vi "GUI_Cameras_v1.2.0.vi"() -> ()   [LabVIEW 2011]
uses:
  <vilib>/Utility/miscctls.llb/LVRectTypeDef.ctl
panel:
  out "Zoom changed":bool
  out "Zoom old":cluster{"X":sgl, "Y":sgl}
  out "MaxCounts":dbl(slide) scale=0.0..256.0
  out "ratio(h)":bool=TRUE
  out "fixsize":bool
  out "Change Ratio":cluster{"X":sgl, "Y":sgl}={"X"=1.6671598, "Y"=0.6151203}
  out "old Panel Bounds":T1={"Left"=105, "Top"=80, "Right"=781, "Bottom"=662}
  in  "shotnumber":i32=354
  in  "gain":dbl
  in  "exposure":dbl=0.52 caption="Exposure"
  in  "save":bool
  in  "trigger":bool
  in  "triggerdelay":dbl
  out "error (h)":bool
  in  "Main Tap":enum32{"IMAQ", "Network", "Internal", "Array"}(tab)
  out "Image (IMAQ)":T2(plugin-control)
  out "local Port":u16=65401
  out "Remote Host":string="192.168.10.157"
  out "port or service name":u16=65400
  in  "timeout ms (slow resp)":i32=500
  in  "reset":bool
  out "All Devices (h)":string[](array[string])
  out "centroidy":dbl
  out "fast ID (h)":refnum<k16>
  out "slow ID (h)":refnum<k16>
  out "error out":errorcluster
  out "connections (hidden)":variant[](array[variant])=[variant(refnum<k16> refnum), variant(refnum<k16> refnum)]
  in  "time to wait (main loop)":i32=200
  in  "time to wait (TCP)":i32=10
  out "Data String":string="exposure,0.520000\r\ntrigger,off\r\nsave,off\r\ngain,0.000000\r\n"
  in  "send":bool
  in  "localsavingpath":path
  out "centroidy":dbl
  out "Image (array)":u8[][](graph)
  out "Device Name (h)":string="FakeCam1"
  out "stop":bool
  out "error message":string
  out "image connection":bool
  out "data connection ok":bool
  # "Data"
  # "Image"
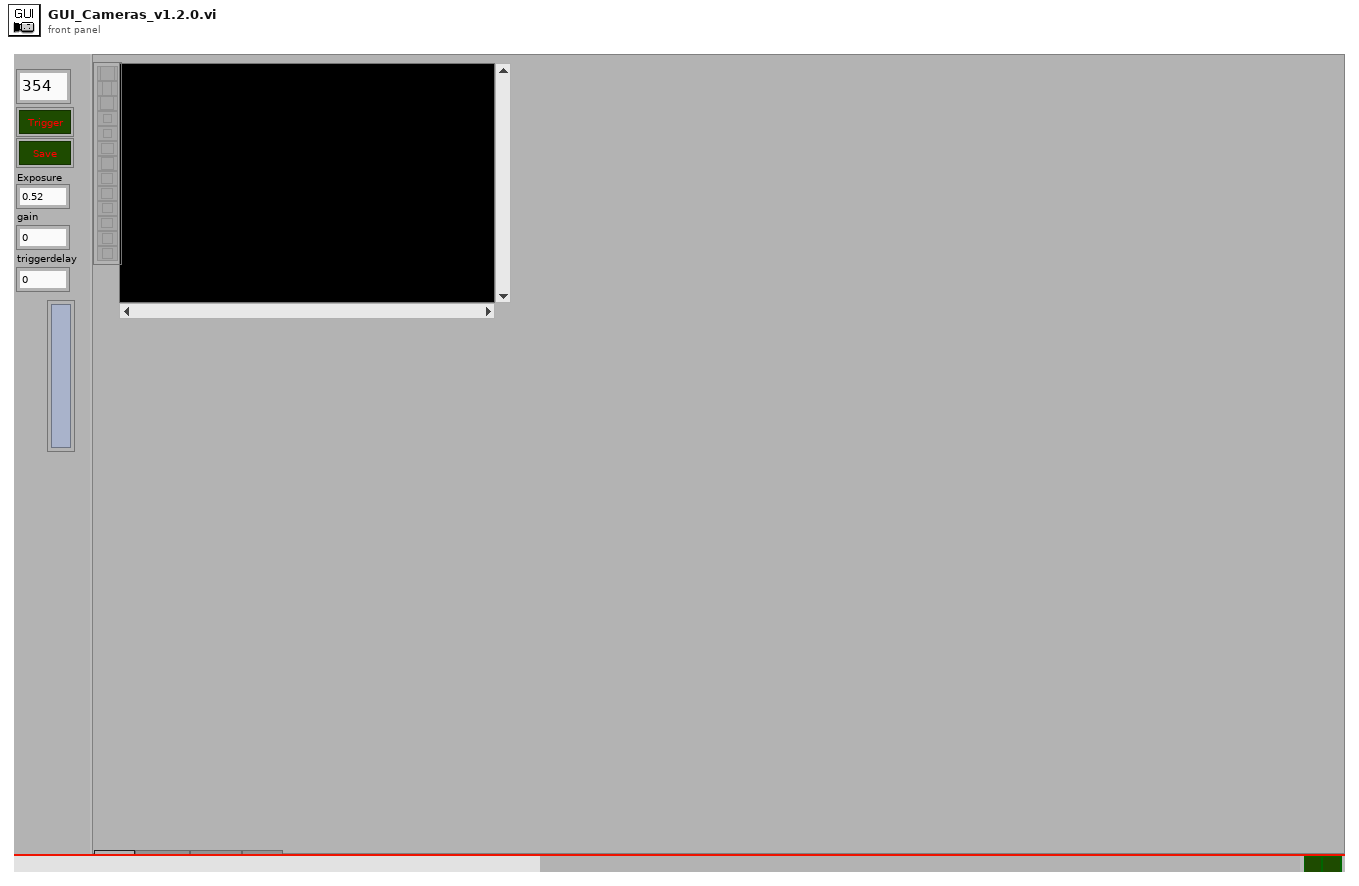
[diagram p1: front panel]
types:
  T1 = typedef "LVRectTypeDef.ctl" = cluster{"Left":i16, "Top":i16, "Right":i16, "Bottom":i16}
  T2 = typedef "IMAQ Image.ctl" = refnum<image>
  T3 = enum16{"Grayscale", "Binary", "Gradient", "Rainbow", "Temperature", "User Defined"}
  T4 = typedef "Image Type" = u32
  T5 = cluster{"Global Rectangle":i32[], "Contours":cluster{"Contour Type":u32, "ROI Type":u32, "Points":i32[]}[]}
  T6 = typedef "ROI Descriptor" = cluster{"Global Rectangle":i32[], "Contours":cluster{"ID":enum32{"External", "Internal"}, "Type":u32, "Coordinates":i32[]}[]}
  T7 = typedef "LVBoundsTypeDef.ctl" = cluster{"Width":u32, "Height":u32}
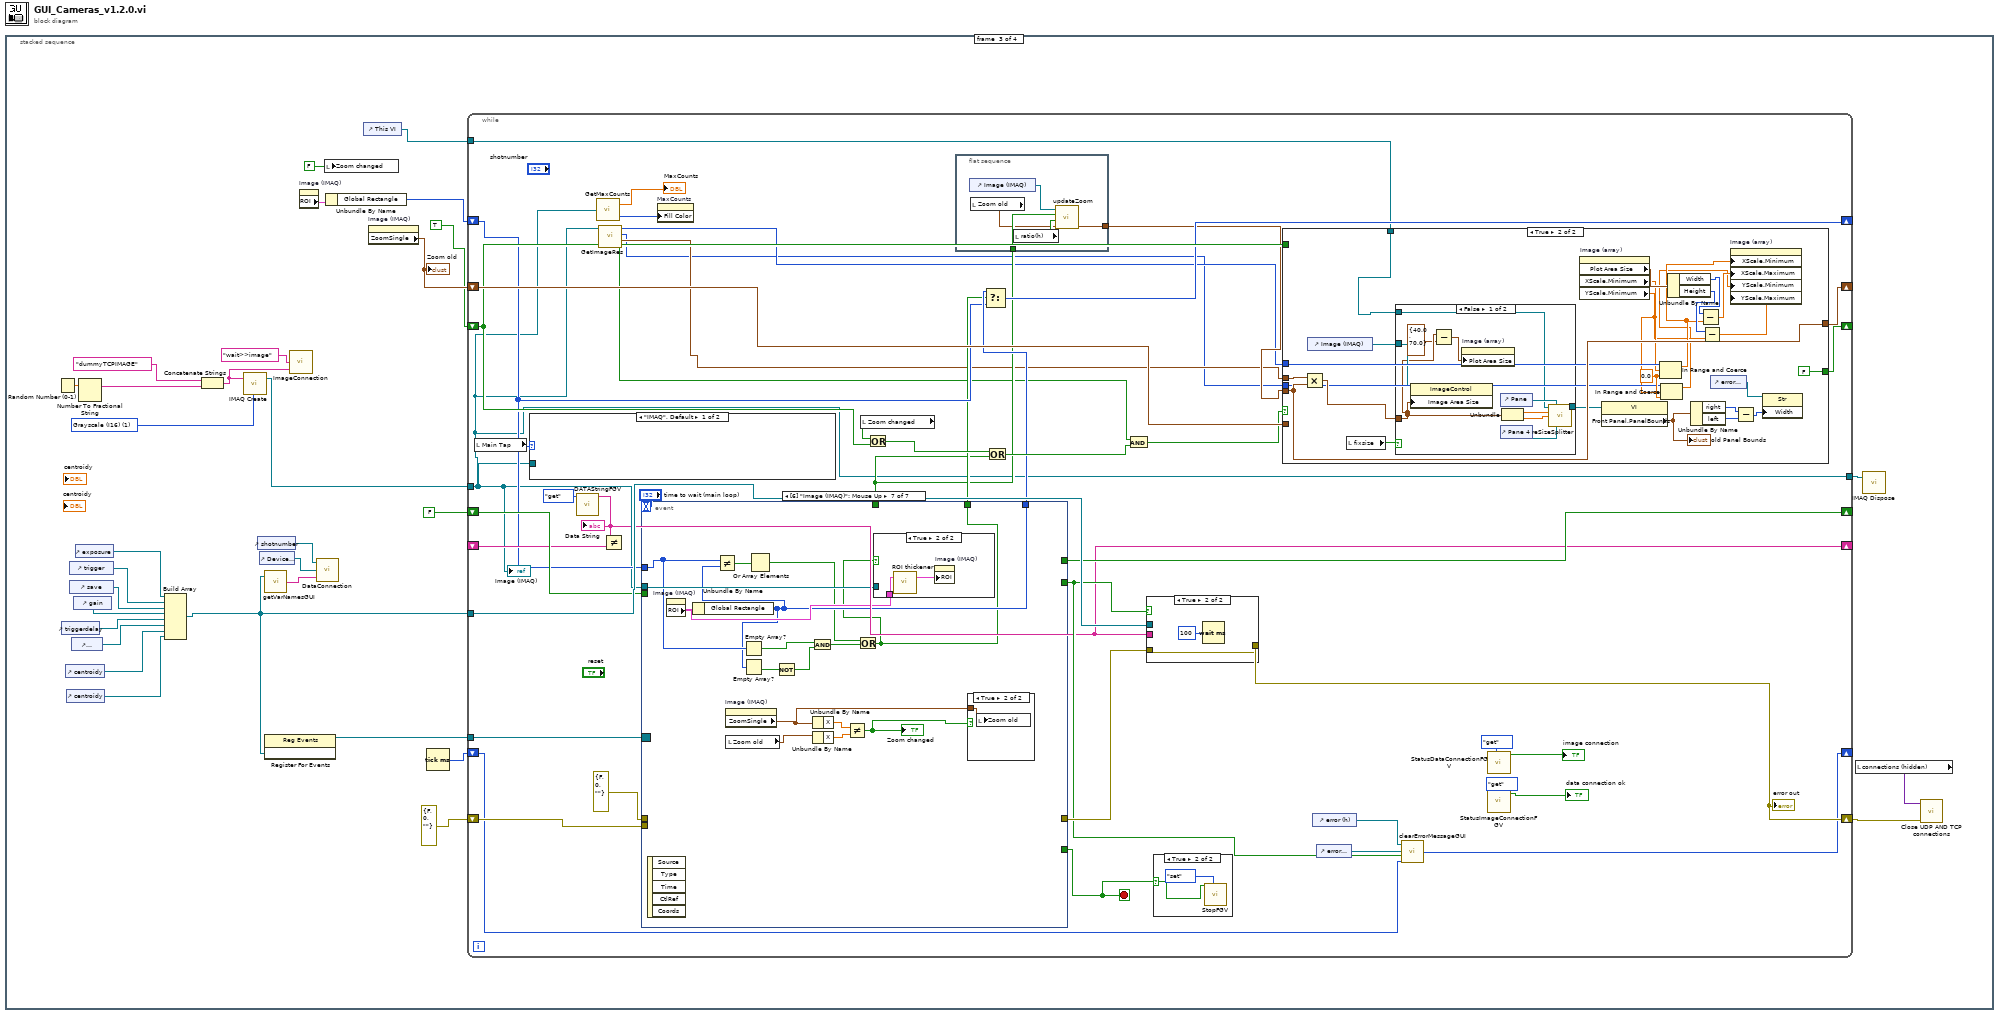
[diagram p0: block diagram]
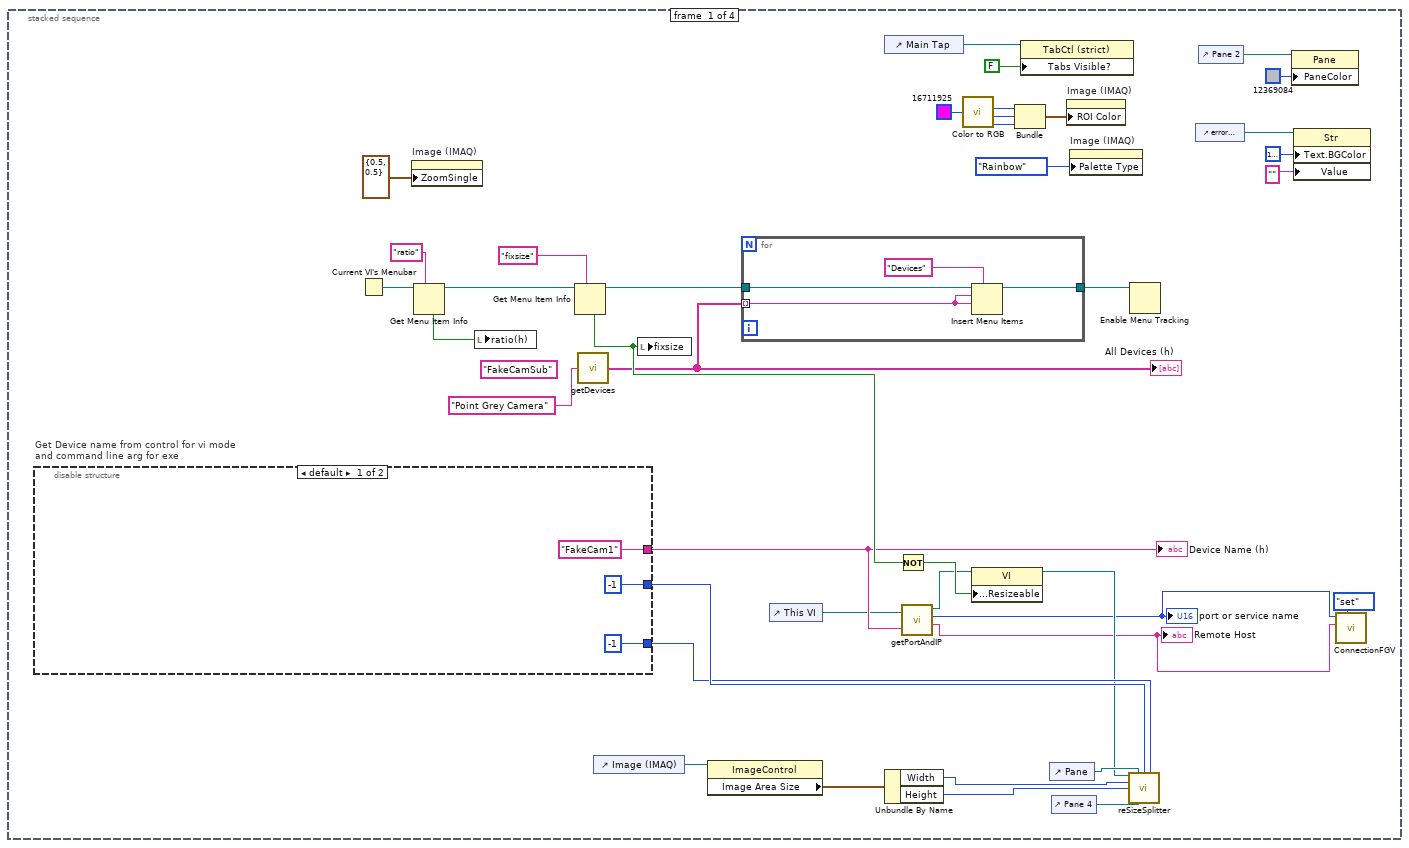
[diagram p2: hidden frame]
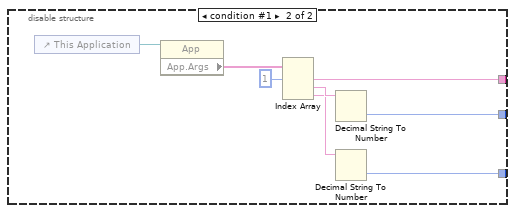
[diagram p3: hidden frame]
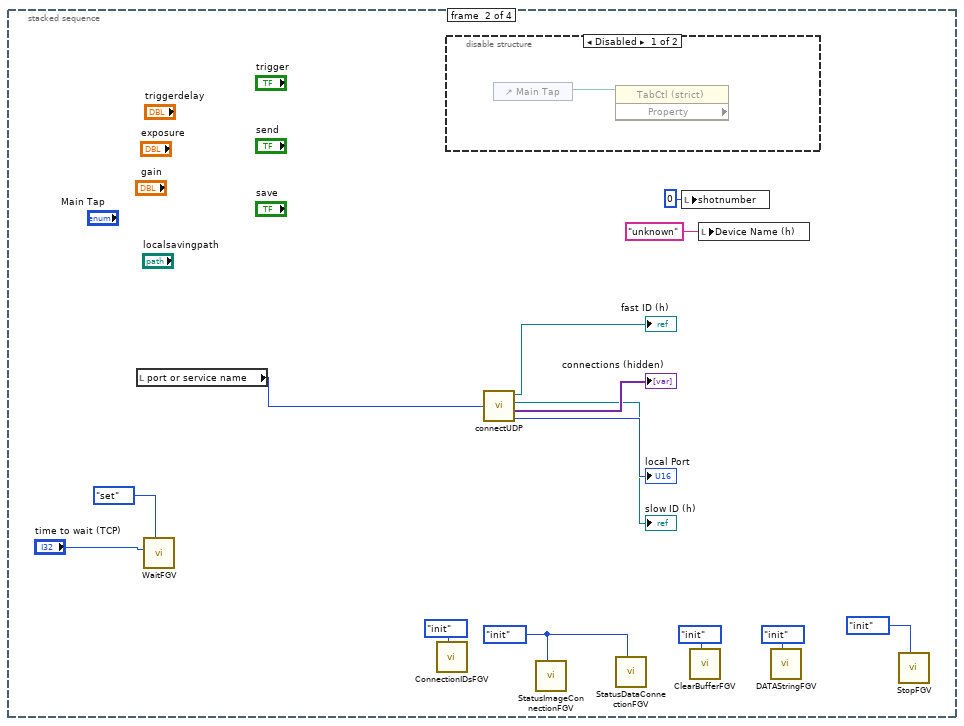
[diagram p4: hidden frame]
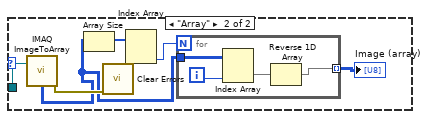
[diagram p7: hidden frame]
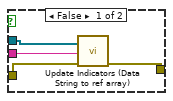
[diagram p10: hidden frame]
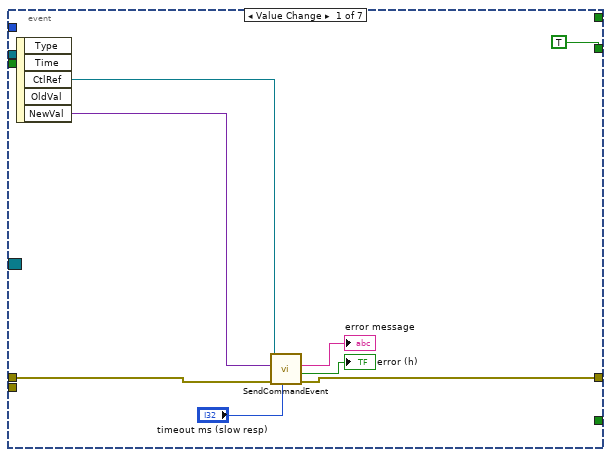
[diagram p11: hidden frame]
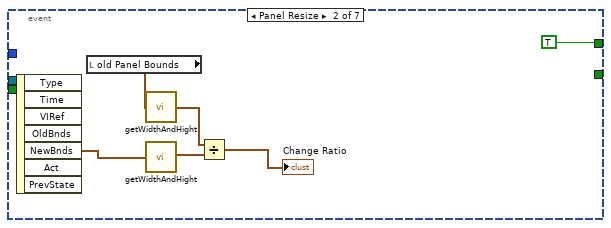
[diagram p12: hidden frame]
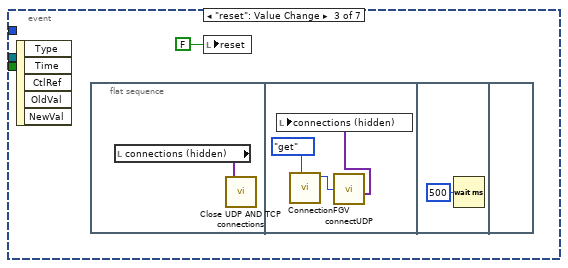
[diagram p13: hidden frame]
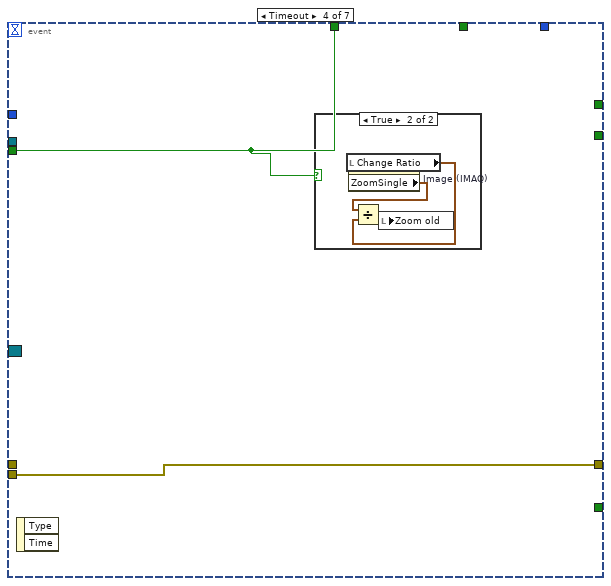
[diagram p14: hidden frame]
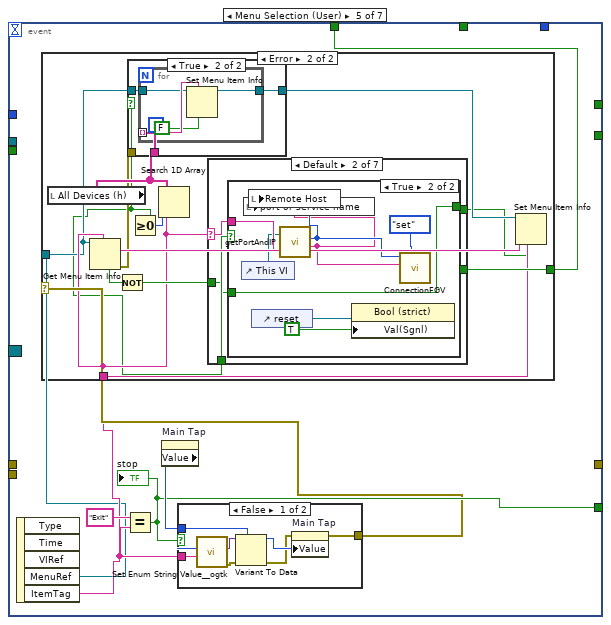
[diagram p16: hidden frame]
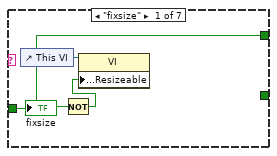
[diagram p19: hidden frame]
diagram:
  n1 = stacked-sequence {
    frame #0 {
      (unwired) "FakeCamSub" ("Device Class")
      n2 = disable-structure "Get Device name from control for vi mode\nand command line arg for exe" shown="default" {
        disable-tunnel: ["FakeCam1" ("Device Name for vi mode") w52] -> w14
        disable-tunnel: [i16 -1 ("left") w49] -> w27
        disable-tunnel: [i16 -1 ("left") w48] -> w26
        frame condition #0 (active) {
        }
        frame condition #1 {
          n3 = control-ref of="This Application"() -> (w55:refnum<vi>)
          n4 = property class="App"(reference=w55) -> ("App.Args"=w54:string[])  [unwired: 1 in, 2 out]
          n5 = Index Array(array=w54, index #1=1 ("index")) -> (element #1=w52:string, element #2=w51:string, element #3=w50:string)  [unwired: 2 in]
          n6 = Decimal String To Number(string=w51) -> (number=w49:i32)  [unwired: 2 in, 1 out]
          n7 = Decimal String To Number(string=w50) -> (number=w48:i32)  [unwired: 2 in, 1 out]
        }
      }
      "Device Name (h)" <- w14
      n8 = Current VI's Menubar() -> (w31:refnum<k9>)
      n9 = property on="Image (IMAQ)" class="ImageControl"("ZoomSingle"=cluster{"X":sgl, "Y":sgl} {"X"=0.5, "Y"=0.5} ("ZoomSingle:All Elements")) -> ()  [unwired: 2 in, 2 out]
      n10 = Get Menu Item Info(7:"ratio" ("item tag"), 11:w31) -> (3:w29:refnum<k9>, 4:w30:bool)  [unwired: 1 in, 5 out]
      n11 = local write "ratio(h)"(w30) -> ()
      n12 = Get Menu Item Info(7:"fixsize" ("item tag"), 11:w29) -> (3:w17:refnum<k9>, 4:w24:bool)  [unwired: 1 in, 5 out]
      n13 = call "getDevices.vi"("Device Class"="Point Grey Camera") -> ("All Devices"=w15:string[])
      "All Devices (h)" <- w15
      n14 = control-ref of="Image (IMAQ)"() -> (w38:refnum<vi>)
      n15 = local write "fixsize"(w24) -> ()
      n16 = property class="ImageControl"(reference=w38) -> ("Image Area Size"=w37:cluster{"Width":u32, "Height":u32})  [unwired: 1 in, 2 out]
      n17 = for {
        tunnel: w17 -> [w44]
        tunnel: [w43] -> w16
        tunnel: w15 -> [w41] mode=indexing
        n18 = Insert Menu Items(5:"Devices" ("menu tag"), 7:w41, 8:w41, 9:w44) -> (3:w43:refnum<k9>)  [unwired: 2 in, 2 out]
      }
      n19 = control-ref of="This VI"() -> (w13:refnum<vi>)
      n20 = control-ref of="Main Tap"() -> (w40:refnum<vi>)
      n21 = Unbundle By Name(w37) -> ("Width"=w36:u32, "Height"=w35:u32)
      n22 = Not(x=w24) -> (.not. x?=w25:bool)
      n23 = call "getPortAndIP.vi"("This Vi"=w13, "Device Name"=w14) -> ("reference out"=w12:refnum<vi>, "port or service name"=w3:u16, "Remote Host"=w2:string)  [unwired: 1 in]
      "port or service name" <- w3
      "Remote Host" <- w2
      n24 = call <vilib>:"Color to RGB.vi"("Color"=u32 16711925) -> ("R"=w9:u8, "G"=w8:u8, "B"=w7:u8)  [unwired: 1 out]
      n25 = property class="VI"(reference=w12, "Front Panel.Resizeable"=w25) -> (reference out=w5:refnum<vi>)  [unwired: 1 in, 1 out]
      n26 = Bundle("R"=w9, "G"=w8, "B"=w7) -> (w6:cluster{"R":u8, "G":u8, "B":u8})  [unwired: 1 in]
      n27 = property class="TabCtl (strict)"(reference=w40, "Tabs Visible?"=FALSE) -> ()  [unwired: 1 in, 2 out]
      n28 = control-ref of="Pane"() -> (w34:refnum<vi>)
      n29 = control-ref of="Pane 4"() -> (w23:refnum<vi>)
      n30 = property on="Image (IMAQ)" class="ImageControl"("ROI Color"=w6) -> ()  [unwired: 2 in, 2 out]
      n31 = property on="Image (IMAQ)" class="ImageControl"("Palette Type"=T3."Rainbow" ("Palette:Palette Type")) -> ()  [unwired: 2 in, 2 out]
      n32 = call "reSizeSplitter.vi"("this vi"=w5, "pane"=w34, "left"=w27, "top"=w26, "Width"=w36, "Height"=w35, "pane2"=w23) -> ()  [unwired: 8 in, 1 out]
      n33 = Enable Menu Tracking(4:w16) -> ()  [unwired: 2 in, 2 out]
      n34 = control-ref of="error message"() -> (w21:refnum<vi>)
      n35 = control-ref of="Pane 2"() -> (w19:refnum<vi>)
      n36 = property class="Pane"(reference=w19, "PaneColor"=u32 12369084) -> ()  [unwired: 1 in, 2 out]
      n37 = property class="Str"(reference=w21, "Text.BGColor"=u32 16777238, "Value"="") -> ()  [unwired: 1 in, 2 out]
      n38 = call "ConnectionFGV.vi"("command"=enum16{"get", "set", "init"}."set", "Remote Host in"=w2, "port or service name in"=w3) -> ()  [unwired: 7 in, 2 out]
    }
    frame #1 {
      w65 = enum16{"get", "set", "init"}."init" ("Command")
      n39 = local read "port or service name"() -> (w67:u16)
      n40 = call "WaitFGV.vi"("Command"=enum16{"get", "set", "init"}."set", "milliseconds to wait"="time to wait (TCP)") -> ()  [unwired: 9 in, 1 out]
      n41 = call "ConnectionIDsFGV.vi"("Command"=enum16{"add", "get", "init"}."init") -> ()  [unwired: 10 in, 1 out]
      n42 = disable-structure shown="Disabled" {
        frame Disabled {
          n43 = control-ref of="Main Tap"() -> (w70:refnum<vi>)
          n44 = property class="TabCtl (strict)" props=[](reference=w70) -> ()  [unwired: 1 in, 3 out]
        }
        frame Enabled {
        }
      }
      n45 = call "connectUDP.vi"("port or service name"=w67) -> ("fast ID (h)"=→"fast ID (h)":refnum<k16>, "slow ID (h)"=→"slow ID (h)":refnum<k16>, "connections (hidden)"=→"connections (hidden)":variant[], "local Port"=→"local Port":u16)
      n46 = call "StatusImageConnectionFGV.vi"("Command"=w65) -> ()  [unwired: 10 in, 1 out]
      n47 = call "StatusDataConnectionFGV.vi"("Command"=w65) -> ()  [unwired: 10 in, 1 out]
      n48 = local write "shotnumber"(0 ("shotnumber")) -> ()
      n49 = call "ClearBufferFGV.vi"("Command"=enum16{"set", "get", "init"}."init") -> ()  [unwired: 10 in, 1 out]
      n50 = local write "Device Name (h)"("unknown" ("Device Name")) -> ()
      n51 = call "DATAStringFGV.vi"("Command"=enum16{"get", "set", "init"}."init") -> ()  [unwired: 10 in, 1 out]
      n52 = call "StopFGV.vi"("Command"=enum16{"set", "get", "init"}."init") -> ()  [unwired: 10 in, 1 out]
    }
    frame #2 {
      w100 = T4 1 items=["Grayscale (U8)", "Grayscale (I16)", "Grayscale (SGL)", "Complex (CSG)", "RGB (U32)", "HSL (U32)", "RGB (U64)", "Grayscale (U16)"] ("Image Type")
      n53 = Random Number (0-1)() -> (number: 0 to 1=w97:dbl)
      n54 = control-ref of="triggerdelay"() -> (w87:refnum<vi>)
      n55 = control-ref of="centroidy"() -> (w81:refnum<vi>)
      n56 = control-ref of="centroidy"() -> (w74:refnum<vi>)
      n57 = control-ref of="trigger"() -> (w91:refnum<vi>)
      n58 = control-ref of="save"() -> (w89:refnum<vi>)
      n59 = control-ref of="localsavingpath"() -> (w82:refnum<vi>)
      n60 = control-ref of="gain"() -> (w88:refnum<vi>)
      n61 = control-ref of="exposure"() -> (w90:refnum<vi>)
      n62 = Number To Fractional String(number=w97) -> (F-format string=w96:string)  [unwired: 3 in]
      n63 = Build Array(w90, w91, w89, w88, w87, w82, w81, w74) -> (w72:refnum<vi>[])
      n64 = Concatenate Strings("dummyTCPIMAGE" ("Image Name"), w96) -> (w94:string)
      n65 = call "IMAQ Create"("Image Name"=w94, "Image Type"=w100) -> ("New Image"=w99:T2)  [unwired: 3 in, 1 out]
      n66 = control-ref of="shotnumber"() -> (w76:refnum<vi>)
      n67 = control-ref of="Device Name (h)"() -> (w75:refnum<vi>)
      n68 = call "getVarNamesGUI.vi"("Array"=w72) -> ("String"=w71:string)  [unwired: 1 in]
      n69 = register-events(w72) -> (reference out=w73:refnum<event-registration>)  [unwired: 2 in, 1 out]
      n70 = call "ImageConnection.vi"("Image Name"=w94, "Image Subscriber list"="wait>>image") -> ()  [unwired: 2 in]
      n71 = property on="Image (IMAQ)" class="ImageControl"() -> ("ROI"=w80:T5)  [unwired: 2 in, 2 out]
      n72 = call "DataConnection.vi"("Subscriber list 2"=w71, "Device Name (h)"=w75, "shotnumber"=w76) -> ()
      n73 = local write "Zoom changed"(FALSE ("Zoom changed")) -> ()
      n74 = Unbundle By Name(w80) -> ("Global Rectangle"=w79:i32[])
      n75 = control-ref of="This VI"() -> (w78:refnum<vi>)
      n76 = property on="Image (IMAQ)" class="ImageControl"() -> ("ZoomSingle"=w86:cluster{"X":sgl, "Y":sgl})  [unwired: 2 in, 2 out]
      "Zoom old" <- w86
      n77 = Tick Count (ms)() -> (millisecond timer value=w83:u32)
      n78 = while {
        shift-right: [w142] -> w98
        shift-left: errorcluster {"status"=FALSE, "code"=0, "source"=""} ("error out") -> [w144]
        tunnel: w99 -> [w116]
        tunnel: [w116] -> w101
        tunnel: w72 -> [w146]
        shift-right: [w141] -> _
        shift-left: w86 -> [w140]
        shift-right: [w138] -> _
        shift-left: FALSE -> [w139]
        shift-right: [w137] -> _
        shift-left: TRUE -> [w136]
        shift-right: [w132] -> _
        shift-left: w83 -> [w131]
        shift-right: [w105] -> _
        shift-left: _ -> [w129]
        shift-right: [w125] -> _
        shift-left: w79 -> [w124]
        tunnel: w78 -> [w122]
        tunnel: w73 -> [w103]
        stop <- w106 stop-if-true
        n79 = local read "Main Tap"() -> (w127:enum32{"IMAQ", "Network", "Internal", "Array"})
        n80 = case shown="\"IMAQ\", Default" w127 {
          tunnel: w116 -> [_ w160]
          frame "IMAQ", Default {
          }
          frame "Array" {
            n81 = call "IMAQ ImageToArray"("Image"=w160) -> ("error out"=w159:errorcluster, "Image Pixels (U8)"=w156:u8[][])  [unwired: 3 in, 3 out]
            n82 = Array Size(array=w156) -> (size(s)=w158:i32[])
            n83 = call <vilib>:"Clear Errors.vi"("error in (no error)"=w159) -> ()  [unwired: 6 in, 1 out]
            n84 = Index Array(array=w158) -> (element #2=w155:i32)  [unwired: 2 in, 1 out]
            n85 = for {
              N: w155 -> [_]
              tunnel: w156 -> [w164]
              tunnel: [w162] -> w157 mode=indexing
              i -> [w161]
              n86 = Index Array(array=w164, index (col)=w161) -> (element=w163:u8[])  [unwired: 1 in]
              n87 = Reverse 1D Array(array=w163) -> (reversed array=w162:u8[])
            }
            "Image (array)" <- w157
          }
        }
        n88 = call "DATAStringFGV.vi"("Command"=enum16{"get", "set", "init"}."get") -> ("Data String out"=w105:string)  [unwired: 10 in]
        "Data String" <- w105
        n89 = call "GetMaxCounts.vi"("New Image"=w116) -> ("Maximal Value"=→"MaxCounts":sgl, "Color"=w118:u32)
        n90 = call "GetImageRes.vi"("Image"=w116) -> ("valid Image"=w114:bool, "Image Area:Size:All Elements"=w115:cluster{"Width":u32, "Height":u32}, "Y Resolution"=w112:i32, "X Resolution"=w113:i32)  [unwired: 7 in]
        n91 = Not Equal?(x=w105, y=w129) -> ()  [unwired: 1 out]
        n92 = event shown="[6] \"Image (IMAQ)\": Mouse Up" {
          selector: w103 -> [_ _ _ _ _ _ _]
          dyn-events: _ -> [_ _ _ _ _ _ _]
          timeout: "time to wait (main loop)" -> [_ _ _ _ _ _ _]
          tunnel: [w214 _ _ w230 _ _ _] -> w143
          tunnel: errorcluster {"status"=FALSE, "code"=0, "source"=""} ("error out") -> [w216 _ _ _ _ _ _]
          tunnel: w144 -> [_ _ _ w230 _ _ _]
          tunnel: [TRUE _ _ _ _ _ _] -> w128
          tunnel: [_ _ _ _ w238 _ _] -> w106
          tunnel: [_ _ _ w229 w235 _ _] -> w121
          tunnel: w139 -> [_ _ _ w229 _ _ _]
          tunnel: [_ TRUE _ _ _ _ _] -> w138
          tunnel: [_ _ _ _ _ _ w316] -> w126
          tunnel: w124 -> [_ _ _ _ _ _ w317]
          tunnel: [_ _ _ _ _ _ w310] -> w123
          tunnel: w116 -> [_ _ _ _ _ _ w319]
          event Value Change {
            n93 = event-data() -> ("CtlRef"=w211:refnum<vi>, "NewVal"=w210:variant)  [unwired: 1 in, 3 out]
            n94 = call "SendCommandEvent.vi"("timeout ms (slow resp)"="timeout ms (slow resp)", "error out 2"=w216, "NewVal"=w210, "CtlRef"=w211) -> ("error out"=w214:errorcluster, "error (h)"=→"error (h)":bool, "error message"=→"error message":string)  [unwired: 4 in, 1 out]
          }
          event Panel Resize {
            n95 = event-data() -> ("NewBnds"=w222:T1)  [unwired: 1 in, 6 out]
            n96 = local read "old Panel Bounds"() -> (w220:T1)
            n97 = call "getWidthAndHight.vi"("OldBnds"=w220) -> ("output cluster"=w219:cluster{"X":sgl, "Y":sgl})
            n98 = call "getWidthAndHight.vi"("OldBnds"=w222) -> ("output cluster"=w218:cluster{"X":sgl, "Y":sgl})
            n99 = Divide(x=w219, y=w218) -> (x/y=→"Change Ratio":cluster{"X":sgl, "Y":sgl})
          }
          event "reset": Value Change {
            n100 = event-data() -> ()  [unwired: 1 in, 5 out]
            n101 = flat-sequence {
              frame #0 {
                n102 = local read "connections (hidden)"() -> (w224:variant[])
                n103 = call "Close UDP AND TCP connections.vi"("appended array"=w224) -> ()  [unwired: 7 in]
              }
              frame #1 {
                n104 = call "ConnectionFGV.vi"("command"=enum16{"get", "set", "init"}."get") -> ("port or service name out"=w226:u16)  [unwired: 9 in, 1 out]
                n105 = call "connectUDP.vi"("port or service name"=w226) -> ("connections (hidden)"=w225:variant[])  [unwired: 3 out]
                n106 = local write "connections (hidden)"(w225) -> ()
              }
              frame #2 {
                n107 = Wait (ms)(milliseconds to wait=u32 500) -> ()  [unwired: 1 out]
              }
              frame #3 {
              }
            }
            n108 = local write "reset"(FALSE ("reset")) -> ()
          }
          event Timeout {
            n109 = event-data() -> ()  [unwired: 1 in, 2 out]
            n110 = case shown="True" w229 {
              frame False {
              }
              frame True {
                n111 = local read "Change Ratio"() -> (w232:cluster{"X":sgl, "Y":sgl})
                n112 = property on="Image (IMAQ)" class="ImageControl"() -> ("ZoomSingle"=w233:cluster{"X":sgl, "Y":sgl})  [unwired: 2 in, 2 out]
                n113 = Divide(x=w233, y=w232) -> (x/y=w231:cluster{"X":sgl, "Y":sgl})
                n114 = local write "Zoom old"(w231) -> ()
              }
            }
          }
          event Menu Selection (User) {
            n115 = event-data() -> ("MenuRef"=w234:refnum<k9>, "ItemTag"=w236:string)  [unwired: 1 in, 3 out]
            n116 = Equal?(x="Exit", y=w236) -> (x = y?=w238:bool)
            "stop" <- w238
            n117 = property on="Main Tap" class="TabCtl (strict)"() -> ("Value"=w240:enum32{"IMAQ", "Network", "Internal", "Array"})  [unwired: 2 in, 2 out]
            n118 = case shown="False" w238 {
              tunnel: w240 -> [w299 _]
              tunnel: w236 -> [w298 _]
              tunnel: [w295 errorcluster {"status"=FALSE, "code"=0, "source"=""} ("error out")] -> w237
              frame False {
                n119 = call <userlib>:"Set Enum String Value__ogtk.vi"("String Value"=w298, "Default Enum Value"=w299) -> ("error out"=w297:errorcluster, "Enum"=w301:variant)  [unwired: 8 in]
                n120 = Variant To Data(error in=w297, type=w299, Variant=w301) -> (data=w300:enum32{"IMAQ", "Network", "Internal", "Array"}, error out=w296:errorcluster)
                n121 = property on="Main Tap" class="TabCtl (strict)"(error in=w296, "Value"=w300) -> (error out=w295:errorcluster)  [unwired: 1 in, 1 out]
              }
              frame True {
              }
            }
            n122 = case shown="Error" w237 {
              tunnel: w234 -> [_ w244]
              tunnel: w236 -> [_ w248]
              tunnel: [_ w249] -> w235
              frame No Error {
              }
              frame Error {
                n123 = local read "All Devices (h)"() -> (w246:string[])
                n124 = Get Menu Item Info(7:w248, 11:w244) -> (0:w245:errorcluster, 2:w251:string, 4:w252:bool)  [unwired: 1 in, 4 out]
                n125 = Not(x=w252) -> (.not. x?=w250:bool)
                n126 = Search 1D Array(1D array=w246, element=w248) -> (index of element=w247:i32)  [unwired: 1 in]
                n127 = Greater Or Equal To 0?(x=w247) -> (x >= 0?=w243:bool)
                n128 = case shown="True" w243 {
                  tunnel: w246 -> [_ w256]
                  tunnel: w245 -> [_ _]
                  tunnel: w244 -> [w253 w255]
                  tunnel: [w253 w254] -> w242
                  frame False {
                  }
                  frame True {
                    n129 = for {
                      tunnel: w256 -> [w260] mode=indexing
                      tunnel: w255 -> [w258]
                      tunnel: [w257] -> w254
                      n130 = Set Menu Item Info(6:FALSE ("checked"), 7:w260, 11:w258) -> (3:w257:refnum<k9>)  [unwired: 4 in, 1 out]
                    }
                  }
                }
                n131 = case shown="Default" w248 {
                  selector: w248 -> [_ w266 _ _ w287 _ _]
                  tunnel: w250 -> [w261 w264 w277 _ _ _ w292]
                  tunnel: [_ _ TRUE _ _ _ _] -> w249
                  tunnel: w243 -> [_ w267 _ _ _ _ _]
                  tunnel: [w261 w265 w277 _ _ _ w292] -> w241
                  frame "fixsize" {
                    n132 = control-ref of="This VI"() -> (w263:refnum<vi>)
                    n133 = Not(x=w261) -> (.not. x?=w262:bool)
                    n134 = property class="VI"(reference=w263, "Front Panel.Resizeable"=w262) -> ()  [unwired: 1 in, 2 out]
                    "fixsize" <- w261
                  }
                  frame Default {
                    n135 = case shown="True" w267 {
                      tunnel: w266 -> [_ w275]
                      tunnel: [_ w271] -> w265
                      tunnel: w264 -> [_ w271]
                      frame False {
                      }
                      frame True {
                        n136 = control-ref of="This VI"() -> (w274:refnum<vi>)
                        n137 = control-ref of="reset"() -> (w273:refnum<vi>)
                        n138 = call "getPortAndIP.vi"("This Vi"=w274, "Device Name"=w275) -> ("port or service name"=w269:u16, "Remote Host"=w268:string)  [unwired: 1 in, 1 out]
                        n139 = local write "port or service name"(w269) -> ()
                        n140 = local write "Remote Host"(w268) -> ()
                        n141 = property class="Bool (strict)"(reference=w273, "Val(Sgnl)"=TRUE ("Value (Signaling)")) -> ()  [unwired: 1 in, 2 out]
                        n142 = call "ConnectionFGV.vi"("command"=enum16{"get", "set", "init"}."set", "Remote Host in"=w268, "port or service name in"=w269) -> ()  [unwired: 7 in, 2 out]
                      }
                    }
                  }
                  frame "ratio" {
                    n143 = property on="Image (IMAQ)" class="ImageControl"() -> ("ZoomSingle"=w276:cluster{"X":sgl, "Y":sgl})  [unwired: 2 in, 2 out]
                    n144 = local write "Zoom old"(w276) -> ()
                    "ratio(h)" <- w277
                  }
                  frame "Local Saving Path" {
                    n145 = control-ref of="localsavingpath"() -> (w279:refnum<vi>)
                    n146 = property class="Path"(reference=w279) -> (reference out=w282:refnum<vi>, "Value"=w283:path)  [unwired: 1 in, 1 out]
                    n147 = call "changePath.vi"("Local Saving in (h)"=w283) -> ("change (h)"=w281:bool, "Local Saving out (h)"=w280:path)  [unwired: 9 in]
                    n148 = case shown="True" w281 {
                      tunnel: w282 -> [_ w285]
                      tunnel: w280 -> [_ w284]
                      frame False {
                      }
                      frame True {
                        n149 = property class="Path"(reference=w285, "Val(Sgnl)"=w284) -> ()  [unwired: 1 in, 2 out]
                      }
                    }
                  }
                  frame "Binary", "Gradient", "Grayscale", "Rainbow", "Temperature" {
                    n150 = Scan From String(input string=w287, default 1=T3."Grayscale" ("Palette:Palette Type")) -> (output 1=w286:T3)  [unwired: 3 in, 3 out]
                    n151 = property on="Image (IMAQ)" class="ImageControl"("Palette Type"=w286) -> ()  [unwired: 2 in, 2 out]
                  }
                  frame "reset" {
                    n152 = control-ref of="reset"() -> (w290:refnum<vi>)
                    n153 = property class="Bool (strict)"(reference=w290, "Val(Sgnl)"=TRUE ("Value (Signaling)")) -> ()  [unwired: 1 in, 2 out]
                  }
                  frame "clear" {
                    n154 = control-ref of="reset"() -> (w294:refnum<vi>)
                    n155 = call "ClearBufferFGV.vi"("Command"=enum16{"set", "get", "init"}."set", "clear buffer"=w292) -> ()  [unwired: 9 in, 1 out]
                    n156 = property class="Bool (strict)"(reference=w294, "Val(Sgnl)"=TRUE ("Value (Signaling)")) -> ()  [unwired: 1 in, 2 out]
                  }
                }
                n157 = Set Menu Item Info(6:w241, 7:w248, 10:w251, 11:w242) -> ()  [unwired: 3 in, 2 out]
              }
            }
          }
          event "time to wait (TCP)": Value Change {
            n158 = event-data() -> ("NewVal"=w304:i32)  [unwired: 1 in, 4 out]
            n159 = call "WaitFGV.vi"("Command"=enum16{"get", "set", "init"}."set", "milliseconds to wait"=w304) -> ()  [unwired: 9 in, 1 out]
          }
          event "Image (IMAQ)": Mouse Up {
            n160 = event-data() -> ()  [unwired: 1 in, 5 out]
            n161 = property on="Image (IMAQ)" class="ImageControl"() -> ("ROI"=w318:T5)  [unwired: 2 in, 2 out]
            n162 = Unbundle By Name(w318) -> ("Global Rectangle"=w316:i32[])
            n163 = Not Equal?(x=w317, y=w316) -> (x != y?=w320:bool[])
            n164 = property on="Image (IMAQ)" class="ImageControl"() -> ("ZoomSingle"=w305:cluster{"X":sgl, "Y":sgl})  [unwired: 2 in, 2 out]
            n165 = local read "Zoom old"() -> (w307:cluster{"X":sgl, "Y":sgl})
            n166 = Empty Array?(array=w317) -> (empty?=w313:bool)
            n167 = Empty Array?(array=w316) -> (empty?=w315:bool)
            n168 = Or Array Elements(Boolean array=w320) -> (logical OR=w311:bool)
            n169 = Not(x=w315) -> (.not. x?=w314:bool)
            n170 = And(x=w313, y=w314) -> (x .and. y?=w312:bool)
            n171 = Unbundle By Name(w305) -> ("X"=w308:sgl)
            n172 = Unbundle By Name(w307) -> ("X"=w309:sgl)
            n173 = Not Equal?(x=w308, y=w309) -> (x != y?=w306:bool)
            "Zoom changed" <- w306
            n174 = Or(x=w311, y=w312) -> (x .or. y?=w310:bool)
            n175 = case shown="True" w310 {
              tunnel: w319 -> [_ _]
              tunnel: w318 -> [_ w323]
              frame False {
              }
              frame True {
                n176 = call "ROI thickener.vi"("ROI Descriptor in"=w323) -> ("ROI Descriptor out"=w322:T6)  [unwired: 1 in, 1 out]
                n177 = property on="Image (IMAQ)" class="ImageControl"("ROI"=w322) -> ()  [unwired: 2 in, 2 out]
              }
            }
            n178 = case shown="True" w306 {
              tunnel: w305 -> [_ w321]
              frame False {
              }
              frame True {
                n179 = local write "Zoom old"(w321) -> ()
              }
            }
          }
        }
        n180 = property on="MaxCounts" class="Slide (strict)"("Fill Color"=w118) -> ()  [unwired: 2 in, 2 out]
        n181 = local read "Zoom changed"() -> (w117:bool)
        n182 = Or(x=w117, y=w136) -> (x .or. y?=w135:bool)
        n183 = flat-sequence {
          tunnel: w121 -> [w153]
          tunnel: [w150] -> w120
          frame #0 {
            n184 = control-ref of="Image (IMAQ)"() -> (w154:refnum<vi>)
            n185 = local read "Zoom old"() -> (w151:cluster{"X":sgl, "Y":sgl})
            n186 = local read "ratio(h)"() -> (w152:bool)
            n187 = call "updateZoom.vi"("Zoom old"=w151, "ratio(h)"=w152, "update Zoom"=w153, "imageRef"=w154) -> ("Zoom out"=w150:cluster{"X":sgl, "Y":sgl})  [unwired: 7 in]
          }
        }
        n188 = Select(t=w126, s=w123, f=w124) -> (s? t:f=w125:i32[])
        n189 = Or(x=w135, y=w121) -> (x .or. y?=w133:bool)
        n190 = And(x=w114, y=w133) -> (x .and. y?=w134:bool)
        n191 = case shown="True" w128 {
          tunnel: w146 -> [w206 _]
          tunnel: w143 -> [w203 w208]
          tunnel: [w205 w208] -> w142
          tunnel: w105 -> [w204 _]
          frame False {
            n192 = call "Update Indicators (Data String to ref array).vi"("Array"=w206, "Data String"=w204, "error in (no error)"=w203) -> ("error out"=w205:errorcluster)  [unwired: 11 in, 1 out]
          }
          frame True {
            n193 = Wait (ms)(milliseconds to wait=u32 100) -> ()  [unwired: 1 out]
          }
        }
        "error out" <- w142
        n194 = case shown="True" w106 {
          selector: w106 -> [_ w148]
          frame False {
          }
          frame True {
            n195 = call "StopFGV.vi"("Command"=enum16{"set", "get", "init"}."set", "Stop"=w148) -> ()  [unwired: 9 in, 1 out]
          }
        }
        n196 = case shown="True" w134 {
          tunnel: w120 -> [_ w190]
          tunnel: [w166 w190] -> w141
          tunnel: w140 -> [w166 _]
          tunnel: w115 -> [_ w191]
          tunnel: w136 -> [w165 _]
          tunnel: [w165 FALSE] -> w137
          tunnel: w113 -> [_ w175]
          tunnel: w112 -> [_ w171]
          tunnel: w122 -> [_ w168]
          frame False {
          }
          frame True {
            w172 = 0.0 ("lower limit")
            n197 = Multiply(x=w191, y=w190) -> (x*y=w189:cluster{sgl, sgl})
            n198 = control-ref of="Image (IMAQ)"() -> (w180:refnum<vi>)
            n199 = local read "fixsize"() -> (w181:bool)
            n200 = case shown="False" w181 {
              tunnel: w189 -> [w194 _]
              tunnel: w168 -> [w198 w202]
              tunnel: [w197 w202] -> w187
              tunnel: w180 -> [w196 _]
              frame False {
                n201 = property class="ImageControl"(reference=w196, "Image Area Size"=w194) -> ()  [unwired: 1 in, 2 out]
                n202 = Subtract(x=w194, y=cluster{sgl, sgl} {40.0, 70.0}) -> (x-y=w193:cluster{sgl, sgl})
                n203 = property on="Image (array)" class="IntGraph (strict)"("Plot Area Size"=w193) -> ()  [unwired: 2 in, 2 out]
                n204 = control-ref of="Pane"() -> (w199:refnum<vi>)
                n205 = control-ref of="Pane 4"() -> (w195:refnum<vi>)
                n206 = Unbundle(w194) -> (w200:sgl, w201:sgl)
                n207 = call "reSizeSplitter.vi"("this vi"=w198, "pane"=w199, "Width"=w200, "Height"=w201, "pane2"=w195) -> ("reference out"=w197:refnum<vi>)  [unwired: 10 in]
              }
              frame True {
              }
            }
            n208 = property on="Image (array)" class="IntGraph (strict)"() -> ("Plot Area Size"=w179:T7, "XScale.Minimum"=w173:dbl, "YScale.Minimum"=w170:dbl)  [unwired: 2 in, 2 out]
            n209 = property class="VI"(reference=w187) -> ("Front Panel.PanelBounds"=w186:T1)  [unwired: 1 in, 2 out]
            "old Panel Bounds" <- w186
            n210 = In Range and Coerce(upper limit=w175, x=w173, lower limit=w172) -> (coerced(x)=w174:dbl)  [unwired: 1 out]
            n211 = In Range and Coerce(upper limit=w171, x=w170, lower limit=w172) -> (coerced(x)=w169:dbl)  [unwired: 1 out]
            n212 = Unbundle By Name(w179) -> ("Width"=w178:u32, "Height"=w176:u32)
            n213 = Unbundle By Name(w186) -> ("right"=w185:i16, "left"=w184:i16)
            n214 = Subtract(x=w178, y=w174) -> (x-y=w177:dbl)
            n215 = Subtract(x=w176, y=w170) -> (x-y=w167:dbl)
            n216 = control-ref of="error message"() -> (w188:refnum<vi>)
            n217 = property on="Image (array)" class="IntGraph (strict)"("XScale.Minimum"=w174, "XScale.Maximum"=w177, "YScale.Minimum"=w169, "YScale.Maximum"=w167) -> ()  [unwired: 2 in, 2 out]
            n218 = Subtract(x=w185, y=w184) -> (x-y=w183:i16)
            n219 = property class="Str"(reference=w188, "Width"=w183) -> ()  [unwired: 1 in, 2 out]
          }
        }
        n220 = control-ref of="error (h)"() -> (w111:refnum<vi>)
        n221 = control-ref of="error message"() -> (w130:refnum<vi>)
        n222 = call "clearErrorMessageGUI.vi"("millisecond timer value"=w131, "Boolean"=w128, "error message"=w130, "reference"=w111) -> ("millisecond timer value 2"=w132:u32)
        n223 = call "StatusDataConnectionFGV.vi"("Command"=enum16{"get", "set", "init"}."get") -> ("Data Connection out"=→"image connection":bool)  [unwired: 10 in]
        n224 = call "StatusImageConnectionFGV.vi"("Command"=enum16{"get", "set", "init"}."get") -> ("Image Connection out"=→"data connection ok":bool)  [unwired: 10 in]
        "Image (IMAQ)" <- w116
      }
      n225 = local read "connections (hidden)"() -> (w93:variant[])
      n226 = call "IMAQ Dispose"("Image"=w101) -> ()  [unwired: 5 in, 1 out]
      n227 = call "Close UDP AND TCP connections.vi"("error in"=w98, "appended array"=w93) -> ()  [unwired: 6 in]
    }
    frame #3 {
      n228 = flat-sequence {
        frame #0 {
          n229 = Wait (ms)(milliseconds to wait=u32 0) -> ()  [unwired: 1 out]
        }
        frame #1 {
          n230 = local write "stop"(FALSE ("stop")) -> ()
        }
        frame #2 {
          n231 = control-ref of="This VI"() -> (w331:refnum<vi>)
          n232 = case shown="True" FALSE {
            tunnel: w331 -> [w332 w335]
            tunnel: [w332 w333] -> w330
            frame False {
            }
            frame True {
              n233 = property class="VI" props=["Front Panel.Open"](reference=w335) -> (reference out=w334:refnum<vi>)  [unwired: 1 in, 2 out]
              n234 = invoke class="VI" method="FP.Close"(reference=w334) -> (reference out=w333:refnum<vi>)  [unwired: 2 in, 2 out]
            }
          }
          n235 = Close Reference(reference=w330) -> ()  [unwired: 1 in, 1 out]
        }
      }
      n236 = control-ref of="Main  Control"() -> (w325:refnum<vi>)
      n237 = property class="TabCtl (strict)"(reference=w325, "Tabs Visible?"=TRUE) -> ()  [unwired: 1 in, 2 out]
      n238 = property class="TabCtl (strict)"(reference=w325, "Tab Location"=enum32{"Top", "Bottom", "Left", "Right"}."Bottom") -> ()  [unwired: 1 in, 2 out]
    }
  }
